vi "ACK.vi"(8 "error in (no error)":errorcluster, 11 "Instrument in":refnum<class "Instrument.lvclass">) -> (0 "error out":errorcluster, 2 "ACK":string, 3 "Instrument out":refnum<class "Instrument.lvclass">)   [LabVIEW 2019, in "Instrument.lvclass"]
uses:
  Instrument.lvclass
  Typedefs/Instrument.Commands--Enum.ctl
  Instrument.lvclass/Instrument.ctl
  bb8a232c-f628-49fe-96b6-aa36c3f8e839.vi
  bb8a232c-f628-49fe-96b6-aa36c3f8e839.vi/51caba6d-6296-446a-a2da-4e263dc9a5d0.vi
  Send and Receive.vi
  bb8a232c-f628-49fe-96b6-aa36c3f8e839.vi/3457157e-31b1-4f4b-a000-bad15da46e63.vi
  Private/Get Client Type.vi
  bb8a232c-f628-49fe-96b6-aa36c3f8e839.vi/51caba6d-6296-446a-a2da-4e263dc9a5d0.vi/f8fdbf53-4149-4752-adf3-b20644714078.vi
  bb8a232c-f628-49fe-96b6-aa36c3f8e839.vi/51caba6d-6296-446a-a2da-4e263dc9a5d0.vi/0b774697-c852-4661-9674-ae8ca0127edb.vi
  bb8a232c-f628-49fe-96b6-aa36c3f8e839.vi/3457157e-31b1-4f4b-a000-bad15da46e63.vi/adaa4b52-e4ac-43a6-8425-a99b309495ef.vi
  bb8a232c-f628-49fe-96b6-aa36c3f8e839.vi/3457157e-31b1-4f4b-a000-bad15da46e63.vi/b3a4f726-081f-43d6-a4f7-6f161f5da339.vi
  bb8a232c-f628-49fe-96b6-aa36c3f8e839.vi/3457157e-31b1-4f4b-a000-bad15da46e63.vi/adaa4b52-e4ac-43a6-8425-a99b309495ef.vi/db8f5dfc-3e2f-450a-b7a8-55384d68e217.vi
  bb8a232c-f628-49fe-96b6-aa36c3f8e839.vi/3457157e-31b1-4f4b-a000-bad15da46e63.vi/adaa4b52-e4ac-43a6-8425-a99b309495ef.vi/be21d635-075e-4d27-9a4f-9885091fc39d.vi
  Private/Get RC Connection Status.vi
  Enum to String.vi
  <userlib>/LevyLab/RemoteControl/API/Send and Receive.vi
  <vilib>/Utility/Data Type/Get Type Information.vi
  <vilib>/JDP Science/JSONtext/JSON text to Variant.vi
  Instrument.GetPublicEvents.vi
  <vilib>/JDP Science/JSONtext/Variant to JSON Text.vi
  <vilib>/National Instruments/GUID Generator/Guid Generator.vi
  Instrument.MessageToProcess.vi
  Private/Instrument.MessageFromProcess.EventStructure.vi
  <vilib>/JDP Science/JSONtext/LVClass Serializer/JSONtext LVClass Serializer.lvclass
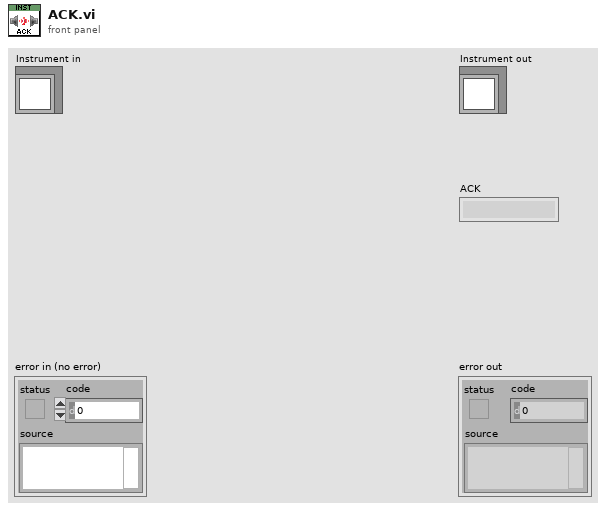
[diagram p1: front panel]
types:
  T1 = typedef "Instrument.lvclass/Instrument.Commands--Enum.ctl" = enum16{"HELP", "ACK", "setConfiguration", "getAll", "getAllData"}
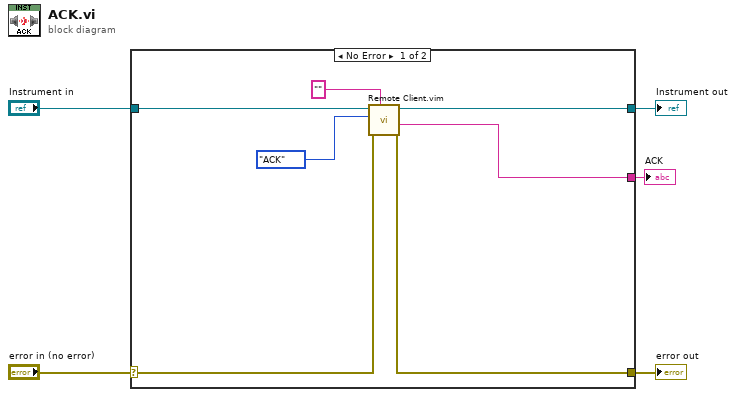
[diagram p0: block diagram]
diagram:
  n1 = case shown="No Error" "error in (no error)" {
    selector: "error in (no error)" -> [w10 w14]
    tunnel: [w7 w14] -> w4
    tunnel: [w12 w13] -> w2
    tunnel: "Instrument in" -> [w11 w13]
    tunnel: [w6 _] -> w1
    frame No Error {
      n2 = call "Remote Client.vim"("Data Out type"="" ("Commands"), "error in (no error)"=w10, "method"=Instrument.Commands--Enum."ACK" ("Commands"), "Instrument in"=w11) -> ("error out"=w7:errorcluster, "Data out"=w6:string, "Instrument out"=w12:refnum<class "Instrument.lvclass">)  [unwired: 4 in, 1 out]
    }
    frame Error {
    }
  }
  "error out" <- w4
  "Instrument out" <- w2
  "ACK" <- w1
